vi "canDataSort.vi"() -> ()   [LabVIEW 2023] (continued)
 8        00\t00\tFF\tFF\tFF\tFF\tFF\tFF\r\n       712  1FFFFFFF   00000004    8        00\t20\tFF\tFF\tFF\tFF\tFF\tFF\r\n       703  0CF102A7   00000004    8        30\t75\tE0\t2E\t80\tFF\tFF\tFD\r\n       744  0CF103A7   00000004    8        17\t1F\t08\t60\tB1\t1F\t08\t3F\r\n       744  0CF102A7   00000004    8        30\t75\tE0\t2E\t80\tFF\tFF\tFD\r\n       743  0C3C4D4A   00000004    8        BE\tFF\tFF\t7F\t18\tFF\tFF\t3F\r\n       743  0CF101A7   00000004    8        68\t00\t97\tCC\t00\t15\t39\t3F\r\n       742  18F120F0   00000004    8        2B\t75\t60\tB1\tB0\t01\tFF\tFF\r\n       741  18F11FF0   00000004    8        FF\t3F\t90\t68\t88\t1B\t10\tFC\r\n       732  1FFFFFFF   00000004    8        00\t20\tFF\tFF\tFF\tFF\tFF\tFF\r\n       723  0CF102A7   00000004    8        30\t75\tE0\t2E\t80\tFF\tFF\tFD\r\n       723  0CF101A7   00000004    8        68\t00\t97\tCC\t00\t15\t39\t3E\r\n       722  1FFFFFFF   00000004    8        00\t00\tFF\tFF\tFF\tFF\tFF\tFF\r\n       712  1FFFFFFF   00000004    8        00\t20\tFF\tFF\tFF\tFF\tFF\tFF\r\n       745  0CF104A7   00000004    8        F0\t60\t22\tFC\tFF\tFF\tFF\t3F\r\n       744  0CF103A7   00000004    8        17\t1F\t08\t60\tB1\t1F\t08\t3F\r\n       744  0CF102A7   00000004    8        30\t75\tE0\t2E\t80\tFF\tFF\tFD\r\n       743  0C3C4D4A   00000004    8        BE\tFF\tFF\t7F\t18\tFF\tFF\t3F\r\n       743  0CF101A7   00000004    8        68\t00\t97\tCC\t00\t15\t39\t3F\r\n       742  18F120F0   00000004    8        2B\t75\t60\tB1\tB0\t01\tFF\tFF\r\n       741  18F11FF0   00000004    8        FF\t3F\t90\t68\t88\t1B\t10\tFC\r\n       732  1FFFFFFF   00000004    8        00\t20\tFF\tFF\tFF\tFF\tFF\tFF\r\n       723  0CF102A7   00000004    8        30\t75\tE0\t2E\t80\tFF\tFF\tFD\r\n       723  0CF101A7   00000004    8        68\t00\t97\tCC\t00\t15\t39\t3E\r\n       722  1FFFFFFF   00000004    8        00\t00\tFF\tFF\tFF\tFF\tFF\tFF\r\n       745  18F106A7   00000004    8        00\tF7\tFF\tFF\tFF\tFF\tFF\t7F\r\n       745  0CF104A7   00000004    8        F0\t60\t22\tFC\tFF\tFF\tFF\t3F\r\n       744  0CF103A7   00000004    8        17\t1F\t08\t60\tB1\t1F\t08\t3F\r\n       744  0CF102A7   00000004    8        30\t75\tE0\t2E\t80\tFF\tFF\tFD\r\n       743  0C3C4D4A   00000004    8        BE\tFF\tFF\t7F\t18\tFF\tFF\t3F\r\n       743  0CF101A7   00000004    8        68\t00\t97\tCC\t00\t15\t39\t3F\r\n       742  18F120F0   00000004    8        2B\t75\t60\tB1\tB0\t01\tFF\tFF\r\n       741  18F11FF0   00000004    8        FF\t3F\t90\t68\t88\t1B\t10\tFC\r\n       732  1FFFFFFF   00000004    8        00\t20\tFF\tFF\tFF\tFF\tFF\tFF\r\n       723  0CF102A7   00000004    8        30\t75\tE0\t2E\t80\tFF\tFF\tFD\r\n       723  0CF101A7   00000004    8        68\t00\t97\tCC\t00\t15\t39\t3E\r\n       746  18F121F0   00000004    8        09\t16\t00\t00\tFF\tFF\tB0\t01\r\n       745  18F106A7   00000004    8        00\tF7\tFF\tFF\tFF\tFF\tFF\t7F\r\n       745  0CF104A7   00000004    8        F0\t60\t22\tFC\tFF\tFF\tFF\t3F\r\n       744  0CF103A7   00000004    8        17\t1F\t08\t60\tB1\t1F\t08\t3F\r\n       744  0CF102A7   00000004    8        30\t75\tE0\t2E\t80\tFF\tFF\tFD\r\n       743  0C3C4D4A   00000004    8        BE\tFF\tFF\t7F\t18\tFF\tFF\t3F\r\n       743  0CF101A7   00000004    8        68\t00\t97\tCC\t00\t15\t39\t3F\r\n       742  18F120F0   00000004    8        2B\t75\t60\tB1\tB0\t01\tFF\tFF\r\n       741  18F11FF0   00000004    8        FF\t3F\t90\t68\t88\t1B\t10\tFC\r\n       732  1FFFFFFF   00000004    8        00\t20\tFF\tFF\tFF\tFF\tFF\tFF\r\n       723  0CF102A7   00000004    8        30\t75\tE0\t2E\t80\tFF\tFF\tFD\r\n       747  1FFFFFFF   00000004    8        00\t20\tFF\tFF\tFF\tFF\tFF\tFF\r\n       746  18F121F0   00000004    8        09\t16\t00\t00\tFF\tFF\tB0\t01\r\n       745  18F106A7   00000004    8        00\tF7\tFF\tFF\tFF\tFF\tFF\t7F\r\n       745  0CF104A7   00000004    8        F0\t60\t22\tFC\tFF\tFF\tFF\t3F\r\n       744  0CF103A7   00000004    8        17\t1F\t08\t60\tB1\t1F\t08\t3F\r\n       744  0CF102A7   00000004    8        30\t75\tE0\t2E\t80\tFF\tFF\tFD\r\n       743  0C3C4D4A   00000004    8        BE\tFF\tFF\t7F\t18\tFF\tFF\t3F\r\n       743  0CF101A7   00000004    8        68\t00\t97\tCC\t00\t15\t39\t3F\r\n       742  18F120F0   00000004    8        2B\t75\t60\tB1\tB0\t01\tFF\tFF\r\n       741  18F11FF0   00000004    8        FF\t3F\t90\t68\t88\t1B\t10\tFC\r\n       732  1FFFFFFF   00000004    8        00\t20\tFF\tFF\tFF\tFF\tFF\tFF\r\n       752  1FFFFFFF   00000004    8        00\t00\tFF\tFF\tFF\tFF\tFF\tFF\r\n       747  1FFFFFFF   00000004    8        00\t20\tFF\tFF\tFF\tFF\tFF\tFF\r\n       746  18F121F0   00000004    8        09\t16\t00\t00\tFF\tFF\tB0\t01\r\n       745  18F106A7   00000004    8        00\tF7\tFF\tFF\tFF\tFF\tFF\t7F\r\n       745  0CF104A7   00000004    8        F0\t60\t22\tFC\tFF\tFF\tFF\t3F\r\n       744  0CF103A7   00000004    8        17\t1F\t08\t60\tB1\t1F\t08\t3F\r\n       744  0CF102A7   00000004    8        30\t75\tE0\t2E\t80\tFF\tFF\tFD\r\n       743  0C3C4D4A   00000004    8        BE\tFF\tFF\t7F\t18\tFF\tFF\t3F\r\n       743  0CF101A7   00000004    8        68\t00\t97\tCC\t00\t15\t39\t3F\r\n       742  18F120F0   00000004    8        2B\t75\t60\tB1\tB0\t01\tFF\tFF\r\n       741  18F11FF0   00000004    8        FF\t3F\t90\t68\t88\t1B\t10\tFC\r\n       762  1FFFFFFF   00000004    8        00\t00\tFF\tFF\tFF\tFF\tFF\tFF\r\n       752  1FFFFFFF   00000004    8        00\t00\tFF\tFF\tFF\tFF\tFF\tFF\r\n       747  1FFFFFFF   00000004    8        00\t20\tFF\tFF\tFF\tFF\tFF\tFF\r\n       746  18F121F0   00000004    8        09\t16\t00\t00\tFF\tFF\tB0\t01\r\n       745  18F106A7   00000004    8        00\tF7\tFF\tFF\tFF\tFF\tFF\t7F\r\n       745  0CF104A7   00000004    8        F0\t60\t22\tFC\tFF\tFF\tFF\t3F\r\n       744  0CF103A7   00000004    8        17\t1F\t08\t60\tB1\t1F\t08\t3F\r\n       744  0CF102A7   00000004    8        30\t75\tE0\t2E\t80\tFF\tFF\tFD\r\n       743  0C3C4D4A   00000004    8        BE\tFF\tFF\t7F\t18\tFF\tFF\t3F\r\n       743  0CF101A7   00000004    8        68\t00\t97\tCC\t00\t15\t39\t3F\r\n       742  18F120F0   00000004    8        2B\t75\t60\tB1\tB0\t01\tFF\tFF\r\n       763  0CF101A7   00000004    8        68\t00\t97\tCC\t00\t15\t39\t40\r\n       762  1FFFFFFF   00000004    8        00\t00\tFF\tFF\tFF\tFF\tFF\tFF\r\n       752  1FFFFFFF   00000004    8        00\t00\tFF\tFF\tFF\tFF\tFF\tFF\r\n       747  1FFFFFFF   00000004    8        00\t20\tFF\tFF\tFF\tFF\tFF\tFF\r\n       746  18F121F0   00000004    8        09\t16\t00\t00\tFF\tFF\tB0\t01\r\n       745  18F106A7   00000004    8        00\tF7\tFF\tFF\tFF\tFF\tFF\t7F\r\n       745  0CF104A7   00000004    8        F0\t60\t22\tFC\tFF\tFF\tFF\t3F\r\n       744  0CF103A7   00000004    8        17\t1F\t08\t60\tB1\t1F\t08\t3F\r\n       744  0CF102A7   00000004    8        30\t75\tE0\t2E\t80\tFF\tFF\tFD\r\n       743  0C3C4D4A   00000004    8        BE\tFF\tFF\t7F\t18\tFF\tFF\t3F\r\n       743  0CF101A7   00000004    8        68\t00\t97\tCC\t00\t15\t39\t3F\r\n       763  0CF102A7   00000004    8        30\t75\tE0\t2E\t80\tFF\tFF\tFD\r\n       763  0CF101A7   00000004    8        68\t00\t97\tCC\t00\t15\t39\t40\r\n       762  1FFFFFFF   00000004    8        00\t00\tFF\tFF\tFF\tFF\tFF\tFF\r\n       752  1FFFFFFF   00000004    8        00\t00\tFF\tFF\tFF\tFF\tFF\tFF\r\n       747  1FFFFFFF   00000004    8        00\t20\tFF\tFF\tFF\tFF\tFF\tFF\r\n       746  18F121F0   00000004    8        09\t16\t00\t00\tFF\tFF\tB0\t01\r\n       745  18F106A7   00000004    8        00\tF7\tFF\tFF\tFF\tFF\tFF\t7F\r\n       745  0CF104A7   00000004    8        F0\t60\t22\tFC\tFF\tFF\tFF\t3F\r\n       744  0CF103A7   00000004    8        17\t1F\t08\t60\tB1\t1F\t08\t3F\r\n       744  0CF102A7   00000004    8        30\t75\tE0\t2E\t80\tFF\tFF\tFD\r\n       743  0C3C4D4A   00000004    8        BE\tFF\tFF\t7F\t18\tFF\tFF\t3F\r\n       772  1FFFFFFF   00000004    8        00\t00\tFF\tFF\tFF\tFF\tFF\tFF\r\n       763  0CF102A7   00000004    8        30\t75\tE0\t2E\t80\tFF\tFF\tFD\r\n       763  0CF101A7   00000004    8        68\t00\t97\tCC\t00\t15\t39\t40\r\n       762  1FFFFFFF   00000004    8        00\t00\tFF\tFF\tFF\tFF\tFF\tFF\r\n       752  1FFFFFFF   00000004    8        00\t00\tFF\tFF\tFF\tFF\tFF\tFF\r\n       747  1FFFFFFF   00000004    8        00\t20\tFF\tFF\tFF\tFF\tFF\tFF\r\n       746  18F121F0   00000004    8        09\t16\t00\t00\tFF\tFF\tB0\t01\r\n       745  18F106A7   00000004    8        00\tF7\tFF\tFF\tFF\tFF\tFF\t7F\r\n       745  0CF104A7   00000004    8        F0\t60\t22\tFC\tFF\tFF\tFF\t3F\r\n       744  0CF103A7   00000004    8        17\t1F\t08\t60\tB1\t1F\t08\t3F\r\n       744  0CF102A7   00000004    8        30\t75\tE0\t2E\t80\tFF\tFF\tFD\r\n       782  1FFFFFFF   00000004    8        00\t00\tFF\tFF\tFF\tFF\tFF\tFF\r\n       772  1FFFFFFF   00000004    8        00\t00\tFF\tFF\tFF\tFF\tFF\tFF\r\n       763  0CF102A7   00000004    8        30\t75\tE0\t2E\t80\tFF\tFF\tFD\r\n       763  0CF101A7   00000004    8        68\t00\t97\tCC\t00\t15\t39\t40\r\n       762  1FFFFFFF   00000004    8        00\t00\tFF\tFF\tFF\tFF\tFF\tFF\r\n       752  1FFFFFFF   00000004    8        00\t00\tFF\tFF\tFF\tFF\tFF\tFF\r\n       747  1FFFFFFF   00000004    8        00\t20\tFF\tFF\tFF\tFF\tFF\tFF\r\n       746  18F121F0   00000004    8        09\t16\t00\t00\tFF\tFF\tB0\t01\r\n       745  18F106A7   00000004    8        00\tF7\tFF\tFF\tFF\tFF\tFF\t7F\r\n       745  0CF104A7   00000004    8        F0\t60\t22\tFC\tFF\tFF\tFF\t3F\r\n       744  0CF103A7   00000004    8        17\t1F\t08\t60\tB1\t1F\t08\t3F\r\n       783  0CF101A7   00000004    8        68\t00\t97\tCC\t00\t15\t39\t41\r\n       782  1FFFFFFF   00000004    8        00\t00\tFF\tFF\tFF\tFF\tFF\tFF\r\n       772  1FFFFFFF   00000004    8        00\t00\tFF\tFF\tFF\tFF\tFF\tFF\r\n       763  0CF102A7   00000004    8        30\t75\tE0\t2E\t80\tFF\tFF\tFD\r\n       763  0CF101A7   00000004    8        68\t00\t97\tCC\t00\t15\t39\t40\r\n       762  1FFFFFFF   00000004    8        00\t00\tFF\tFF\tFF\tFF\tFF\tFF\r\n       752  1FFFFFFF   00000004    8        00\t00\tFF\tFF\tFF\tFF\tFF\tFF\r\n       747  1FFFFFFF   00000004    8        00\t20\tFF\tFF\tFF\tFF\tFF\tFF\r\n       746  18F121F0   00000004    8        09\t16\t00\t00\tFF\tFF\tB0\t01\r\n       745  18F106A7   00000004    8        00\tF7\tFF\tFF\tFF\tFF\tFF\t7F\r\n       745  0CF104A7   00000004    8        F0\t60\t22\tFC\tFF\tFF\tFF\t3F\r\n       783  0CF102A7   00000004    8        30\t75\tE0\t2E\t80\tFF\tFF\tFD\r\n       783  0CF101A7   00000004    8        68\t00\t97\tCC\t00\t15\t39\t41\r\n       782  1FFFFFFF   00000004    8        00\t00\tFF\tFF\tFF\tFF\tFF\tFF\r\n       772  1FFFFFFF   00000004    8        00\t00\tFF\tFF\tFF\tFF\tFF\tFF\r\n       763  0CF102A7   00000004    8        30\t75\tE0\t2E\t80\tFF\tFF\tFD\r\n       763  0CF101A7   00000004    8        68\t00\t97\tCC\t00\t15\t39\t40\r\n       762  1FFFFFFF   00000004    8        00\t00\tFF\tFF\tFF\tFF\tFF\tFF\r\n       752  1FFFFFFF   00000004    8        00\t00\tFF\tFF\tFF\tFF\tFF\tFF\r\n       747  1FFFFFFF   00000004    8        00\t20\tFF\tFF\tFF\tFF\tFF\tFF\r\n       746  18F121F0   00000004    8        09\t16\t00\t00\tFF\tFF\tB0\t01\r\n       745  18F106A7   00000004    8        00\tF7\tFF\tFF\tFF\tFF\tFF\t7F\r\n       792  1FFFFFFF   00000004    8        00\t20\tFF\tFF\tFF\tFF\tFF\tFF\r\n       783  0CF102A7   00000004    8        30\t75\tE0\t2E\t80\tFF\tFF\tFD\r\n       783  0CF101A7   00000004    8        68\t00\t97\tCC\t00\t15\t39\t41\r\n       782  1FFFFFFF   00000004    8        00\t00\tFF\tFF\tFF\tFF\tFF\tFF\r\n       772  1FFFFFFF   00000004    8        00\t00\tFF\tFF\tFF\tFF\tFF\tFF\r\n       763  0CF102A7   00000004    8        30\t75\tE0\t2E\t80\tFF\tFF\tFD\r\n       763  0CF101A7   00000004    8        68\t00\t97\tCC\t00\t15\t39\t40\r\n       762  1FFFFFFF   00000004    8        00\t00\tFF\tFF\tFF\tFF\tFF\tFF\r\n       752  1FFFFFFF   00000004    8        00\t00\tFF\tFF\tFF\tFF\tFF\tFF\r\n       747  1FFFFFFF   00000004    8        00\t20\tFF\tFF\tFF\tFF\tFF\tFF\r\n       746  18F121F0   00000004    8        09\t16\t00\t00\tFF\tFF\tB0\t01\r\n       793  18F106A7   00000004    8        00\tF7\tFF\tFF\tFF\tFF\tFF\t80\r\n       792  1FFFFFFF   00000004    8        00\t20\tFF\tFF\tFF\tFF\tFF\tFF\r\n       783  0CF102A7   00000004    8        30\t75\tE0\t2E\t80\tFF\tFF\tFD\r\n       783  0CF101A7   00000004    8        68\t00\t97\tCC\t00\t15\t39\t41\r\n       782  1FFFFFFF   00000004    8        00\t00\tFF\tFF\tFF\tFF\tFF\tFF\r\n       772  1FFFFFFF   00000004    8        00\t00\tFF\tFF\tFF\tFF\tFF\tFF\r\n       763  0CF102A7   00000004    8        30\t75\tE0\t2E\t80\tFF\tFF\tFD\r\n       763  0CF101A7   00000004    8        68\t00\t97\tCC\t00\t15\t39\t40\r\n       762  1FFFFFFF   00000004    8        00\t00\tFF\tFF\tFF\tFF\tFF\tFF\r\n       752  1FFFFFFF   00000004    8        00\t00\tFF\tFF\tFF\tFF\tFF\tFF\r\n       747  1FFFFFFF   00000004    8        00\t20\tFF\tFF\tFF\tFF\tFF\tFF\r\n       802  1FFFFFFF   00000004    8        00\t20\tFF\tFF\tFF\tFF\tFF\tFF\r\n       793  18F106A7   00000004    8        00\tF7\tFF\tFF\tFF\tFF\tFF\t80\r\n       792  1FFFFFFF   00000004    8        00\t20\tFF\tFF\tFF\tFF\tFF\tFF\r\n       783  0CF102A7   00000004    8        30\t75\tE0\t2E\t80\tFF\tFF\tFD\r\n       783  0CF101A7   00000004    8        68\t00\t97\tCC\t00\t15\t39\t41\r\n       782  1FFFFFFF   00000004    8        00\t00\tFF\tFF\tFF\tFF\tFF\tFF\r\n       772  1FFFFFFF   00000004    8        00\t00\tFF\tFF\tFF\tFF\tFF\tFF\r\n       763  0CF102A7   00000004    8        30\t75\tE0\t2E\t80\tFF\tFF\tFD\r\n       763  0CF101A7   00000004    8        68\t00\t97\tCC\t00\t15\t39\t40\r\n       762  1FFFFFFF   00000004    8        00\t00\tFF\tFF\tFF\tFF\tFF\tFF\r\n       752  1FFFFFFF   00000004    8        00\t00\tFF\tFF\tFF\tFF\tFF\tFF\r\n       803  0CF101A7   00000004    8        68\t00\t97\tCC\t00\t15\t39\t42\r\n       802  1FFFFFFF   00000004    8        00\t20\tFF\tFF\tFF\tFF\tFF\tFF\r\n       793  18F106A7   00000004    8        00\tF7\tFF\tFF\tFF\tFF\tFF\t80\r\n       792  1FFFFFFF   00000004    8        00\t20\tFF\tFF\tFF\tFF\tFF\tFF\r\n       783  0CF102A7   00000004    8        30\t75\tE0\t2E\t80\tFF\tFF\tFD\r\n       783  0CF101A7   00000004    8        68\t00\t97\tCC\t00\t15\t39\t41\r\n       782  1FFFFFFF   00000004    8        00\t00\tFF\tFF\tFF\tFF\tFF\tFF\r\n       772  1FFFFFFF   00000004    8        00\t00\tFF\tFF\tFF\tFF\tFF\tFF\r\n       763  0CF102A7   00000004    8        30\t75\tE0\t2E\t80\tFF\tFF\tFD\r\n       763  0CF101A7   00000004    8        68\t00\t97\tCC\t00\t15\t39\t40\r\n       762  1FFFFFFF   00000004    8        00\t00\tFF\tFF\tFF\tFF\tFF\tFF\r\n       803  0CF102A7   00000004    8        30\t75\tE0\t2E\t80\tFF\tFF\tFD\r\n       803  0CF101A7   00000004    8        68\t00\t97\tCC\t00\t15\t39\t42\r\n       802  1FFFFFFF   00000004    8        00\t20\tFF\tFF\tFF\tFF\tFF\tFF\r\n       793  18F106A7   00000004    8        00\tF7\tFF\tFF\tFF\tFF\tFF\t80\r\n       792  1FFFFFFF   00000004    8        00\t20\tFF\tFF\tFF\tFF\tFF\tFF\r\n       783  0CF102A7   00000004    8        30\t75\tE0\t2E\t80\tFF\tFF\tFD\r\n       783  0CF101A7   00000004    8        68\t00\t97\tCC\t00\t15\t39\t41\r\n       782  1FFFFFFF   00000004    8        00\t00\tFF\tFF\tFF\tFF\tFF\tFF\r\n       772  1FFFFFFF   00000004    8        00\t00\tFF\tFF\tFF\tFF\tFF\tFF\r\n       763  0CF102A7   00000004    8        30\t75\tE0\t2E\t80\tFF\tFF\tFD\r\n       763  0CF101A7   00000004    8        68\t00\t97\tCC\t00\t15\t39\t40\r\n       812  1FFFFFFF   00000004    8        00\t00\tFF\tFF\tFF\tFF\tFF\tFF\r\n       803  0CF102A7   00000004    8        30\t75\tE0\t2E\t80\tFF\tFF\tFD\r\n       803  0CF101A7   00000004    8        68\t00\t97\tCC\t00\t15\t39\t42\r\n       802  1FFFFFFF   00000004    8        00\t20\tFF\tFF\tFF\tFF\tFF\tFF\r\n       793  18F106A7   00000004    8        00\tF7\tFF\tFF\tFF\tFF\tFF\t80\r\n       792  1FFFFFFF   00000004    8        00\t20\tFF\tFF\tFF\tFF\tFF\tFF\r\n       783  0CF102A7   00000004    8        30\t75\tE0\t2E\t80\tFF\tFF\tFD\r\n       783  0CF101A7   00000004    8        68\t00\t97\tCC\t00\t15\t39\t41\r\n       782  1FFFFFFF   00000004    8        00\t00\tFF\tFF\tFF\tFF\tFF\tFF\r\n       772  1FFFFFFF   00000004    8        00\t00\tFF\tFF\tFF\tFF\tFF\tFF\r\n       763  0CF102A7   00000004    8        30\t75\tE0\t2E\t80\tFF\tFF\tFD\r\n       822  1FFFFFFF   00000004    8        00\t00\tFF\tFF\tFF\tFF\tFF\tFF\r\n       812  1FFFFFFF   00000004    8        00\t00\tFF\tFF\tFF\tFF\tFF\tFF\r\n       803  0CF102A7   00000004    8        30\t75\tE0\t2E\t80\tFF\tFF\tFD\r\n       803  0CF101A7   00000004    8        68\t00\t97\tCC\t00\t15\t39\t42\r\n       802  1FFFFFFF   00000004    8        00\t20\tFF\tFF\tFF\tFF\tFF\tFF\r\n       793  18F106A7   00000004    8        00\tF7\tFF\tFF\tFF\tFF\tFF\t80\r\n       792  1FFFFFFF   00000004    8        00\t20\tFF\tFF\tFF\tFF\tFF\tFF\r\n       783  0CF102A7   00000004    8        30\t75\tE0\t2E\t80\tFF\tFF\tFD\r\n       783  0CF101A7   00000004    8        68\t00\t97\tCC\t00\t15\t39\t41\r\n       782  1FFFFFFF   00000004    8        00\t00\tFF\tFF\tFF\tFF\tFF\tFF\r\n       772  1FFFFFFF   00000004    8        00\t00\tFF\tFF\tFF\tFF\tFF\tFF\r\n       823  0CF101A7   00000004    8        68\t00\t97\tCC\t00\t15\t39\t43\r\n       822  1FFFFFFF   00000004    8        00\t00\tFF\tFF\tFF\tFF\tFF\tFF\r\n       812  1FFFFFFF   00000004    8        00\t00\tFF\tFF\tFF\tFF\tFF\tFF\r\n       803  0CF102A7   00000004    8        30\t75\tE0\t2E\t80\tFF\tFF\tFD\r\n       803  0CF101A7   00000004    8        68\t00\t97\tCC\t00\t15\t39\t42\r\n       802  1FFFFFFF   00000004    8        00\t20\tFF\tFF\tFF\tFF\tFF\tFF\r\n       793  18F106A7   00000004    8        00\tF7\tFF\tFF\tFF\tFF\tFF\t80\r\n       792  1FFFFFFF   00000004    8        00\t20\tFF\tFF\tFF\tFF\tFF\tFF\r\n       783  0CF102A7   00000004    8        30\t75\tE0\t2E\t80\tFF\tFF\tFD\r\n       783  0CF101A7   00000004    8        68\t00\t97\tCC\t00\t15\t39\t41\r\n       782  1FFFFFFF   00000004    8        00\t00\tFF\tFF\tFF\tFF\tFF\tFF\r\n       823  0CF102A7   00000004    8        30\t75\tE0\t2E\t80\tFF\tFF\tFD\r\n       823  0CF101A7   00000004    8        68\t00\t97\tCC\t00\t15\t39\t43\r\n       822  1FFFFFFF   00000004    8        00\t00\tFF\tFF\tFF\tFF\tFF\tFF\r\n       812  1FFFFFFF   00000004    8        00\t00\tFF\tFF\tFF\tFF\tFF\tFF\r\n       803  0CF102A7   00000004    8        30\t75\tE0\t2E\t80\tFF\tFF\tFD\r\n       803  0CF101A7   00000004    8        68\t00\t97\tCC\t00\t15\t39\t42\r\n       802  1FFFFFFF   00000004    8        00\t20\tFF\tFF\tFF\tFF\tFF\tFF\r\n       793  18F106A7   00000004    8        00\tF7\tFF\tFF\tFF\tFF\tFF\t80\r\n       792  1FFFFFFF   00000004    8        00\t20\tFF\tFF\tFF\tFF\tFF\tFF\r\n       783  0CF102A7   00000004    8        30\t75\tE0\t2E\t80\tFF\tFF\tFD\r\n       783  0CF101A7   00000004    8        68\t00\t97\tCC\t00\t15\t39\t41\r\n       832  1FFFFFFF   00000004    8        00\t00\tFF\tFF\tFF\tFF\tFF\tFF\r\n       823  0CF102A7   00000004    8        30\t75\tE0\t2E\t80\tFF\tFF\tFD\r\n       823  0CF101A7   00000004    8        68\t00\t97\tCC\t00\t15\t39\t43\r\n       822  1FFFFFFF   00000004    8        00\t00\tFF\tFF\tFF\tFF\tFF\tFF\r\n       812  1FFFFFFF   00000004    8        00\t00\tFF\tFF\tFF\tFF\tFF\tFF\r\n       803  0CF102A7   00000004    8        30\t75\tE0\t2E\t80\tFF\tFF\tFD\r\n       803  0CF101A7   00000004    8        68\t00\t97\tCC\t00\t15\t39\t42\r\n       802  1FFFFFFF   00000004    8        00\t20\tFF\tFF\tFF\tFF\tFF\tFF\r\n       793  18F106A7   00000004    8        00\tF7\tFF\tFF\tFF\tFF\tFF\t80\r\n       792  1FFFFFFF   00000004    8        00\t20\tFF\tFF\tFF\tFF\tFF\tFF\r\n       783  0CF102A7   00000004    8        30\t75\tE0\t2E\t80\tFF\tFF\tFD\r\n       841  18F11FF0   00000004    8        FF\t3F\t90\t68\t88\t1B\t10\t0C\r\n       832  1FFFFFFF   00000004    8        00\t00\tFF\tFF\tFF\tFF\tFF\tFF\r\n       823  0CF102A7   00000004    8        30\t75\tE0\t2E\t80\tFF\tFF\tFD\r\n       823  0CF101A7   00000004    8        68\t00\t97\tCC\t00\t15\t39\t43\r\n       822  1FFFFFFF   00000004    8        00\t00\tFF\tFF\tFF\tFF\tFF\tFF\r\n       812  1FFFFFFF   00000004    8        00\t00\tFF\tFF\tFF\tFF\tFF\tFF\r\n       803  0CF102A7   00000004    8        30\t75\tE0\t2E\t80\tFF\tFF\tFD\r\n       803  0CF101A7   00000004    8        68\t00\t97\tCC\t00\t15\t39\t42\r\n       802  1FFFFFFF   00000004    8        00\t20\tFF\tFF\tFF\tFF\tFF\tFF\r\n       793  18F106A7   00000004    8        00\tF7\tFF\tFF\tFF\tFF\tFF\t80\r\n       792  1FFFFFFF   00000004    8        00\t20\tFF\tFF\tFF\tFF\tFF\tFF\r\n       842  18F120F0   00000004    8        2B\t75\t60\tB1\tB0\t01\tFF\tFF\r\n       841  18F11FF0   00000004    8        FF\t3F\t90\t68\t88\t1B\t10\t0C\r\n       832  1FFFFFFF   00000004    8        00\t00\tFF\tFF\tFF\tFF\tFF\tFF\r\n       823  0CF102A7   00000004    8        30\t75\tE0\t2E\t80\tFF\tFF\tFD\r\n       823  0CF101A7   00000004    8        68\t00\t97\tCC\t00\t15\t39\t43\r\n       822  1FFFFFFF   00000004    8        00\t00\tFF\tFF\tFF\tFF\tFF\tFF\r\n       812  1FFFFFFF   00000004    8        00\t00\tFF\tFF\tFF\tFF\tFF\tFF\r\n       803  0CF102A7   00000004    8        30\t75\tE0\t2E\t80\tFF\tFF\tFD\r\n       803  0CF101A7   00000004    8        68\t00\t97\tCC\t00\t15\t39\t42\r\n       802  1FFFFFFF   00000004    8        00\t20\tFF\tFF\tFF\tFF\tFF\tFF\r\n       793  18F106A7   00000004    8        00\tF7\tFF\tFF\tFF\tFF\tFF\t80\r\n       843  0CF101A7   00000004    8        68\t00\t97\tCC\t00\t15\t39\t44\r\n       842  18F120F0   00000004    8        2B\t75\t60\tB1\tB0\t01\tFF\tFF\r\n       841  18F11FF0   00000004    8        FF\t3F\t90\t68\t88\t1B\t10\t0C\r\n       832  1FFFFFFF   00000004    8        00\t00\tFF\tFF\tFF\tFF\tFF\tFF\r\n       823  0CF102A7   00000004    8        30\t75\tE0\t2E\t80\tFF\tFF\tFD\r\n       823  0CF101A7   00000004    8        68\t00\t97\tCC\t00\t15\t39\t43\r\n       822  1FFFFFFF   00000004    8        00\t00\tFF\tFF\tFF\tFF\tFF\tFF\r\n       812  1FFFFFFF   00000004    8        00\t00\tFF\tFF\tFF\tFF\tFF\tFF\r\n       803  0CF102A7   00000004    8        30\t75\tE0\t2E\t80\tFF\tFF\tFD\r\n       803  0CF101A7   00000004    8        68\t00\t97\tCC\t00\t15\t39\t42\r\n       802  1FFFFFFF   00000004    8        00\t20\tFF\tFF\tFF\tFF\tFF\tFF\r\n       843  0C3C4D4A   00000004    8        BE\tFF\tFF\t7F\t18\tFF\tFF\t40\r\n       843  0CF101A7   00000004    8        68\t00\t97\tCC\t00\t15\t39\t44\r\n       842  18F120F0   00000004    8        2B\t75\t60\tB1\tB0\t01\tFF\tFF\r\n       841  18F11FF0   00000004    8        FF\t3F\t90\t68\t88\t1B\t10\t0C\r\n       832  1FFFFFFF   00000004    8        00\t00\tFF\tFF\tFF\tFF\tFF\tFF\r\n       823  0CF102A7   00000004    8        30\t75\tE0\t2E\t80\tFF\tFF\tFD\r\n       823  0CF101A7   00000004    8        68\t00\t97\tCC\t00\t15\t39\t43\r\n       822  1FFFFFFF   00000004    8        00\t00\tFF\tFF\tFF\tFF\tFF\tFF\r\n       812  1FFFFFFF   00000004    8        00\t00\tFF\tFF\tFF\tFF\tFF\tFF\r\n       803  0CF102A7   00000004    8        30\t75\tE0\t2E\t80\tFF\tFF\tFD\r\n       803  0CF101A7   00000004    8        68\t00\t97\tCC\t00\t15\t39\t42\r\n       844  0CF102A7   00000004    8        30\t75\tE0\t2E\t80\tFF\tFF\tFD\r\n       843  0C3C4D4A   00000004    8        BE\tFF\tFF\t7F\t18\tFF\tFF\t40\r\n       843  0CF101A7   00000004    8        68\t00\t97\tCC\t00\t15\t39\t44\r\n       842  18F120F0   00000004    8        2B\t75\t60\tB1\tB0\t01\tFF\tFF\r\n       841  18F11FF0   00000004    8        FF\t3F\t90\t68\t88\t1B\t10\t0C\r\n       832  1FFFFFFF   00000004    8        00\t00\tFF\tFF\tFF\tFF\tFF\tFF\r\n       823  0CF102A7   00000004    8        30\t75\tE0\t2E\t80\tFF\tFF\tFD\r\n       823  0CF101A7   00000004    8        68\t00\t97\tCC\t00\t15\t39\t43\r\n       822  1FFFFFFF   00000004    8        00\t00\tFF\tFF\tFF\tFF\tFF\tFF\r\n       812  1FFFFFFF   00000004    8        00\t00\tFF\tFF\tFF\tFF\tFF\tFF\r\n       803  0CF102A7   00000004    8        30\t75\tE0\t2E\t80\tFF\tFF\tFD\r\n       844  0CF103A7   00000004    8        17\t1F\t08\t60\tB1\t1F\t08\t40\r\n       844  0CF102A7   00000004    8        30\t75\tE0\t2E\t80\tFF\tFF\tFD\r\n       843  0C3C4D4A   00000004    8        BE\tFF\tFF\t7F\t18\tFF\tFF\t40\r\n       843  0CF101A7   00000004    8        68\t00\t97\tCC\t00\t15\t39\t44\r\n       842  18F120F0   00000004    8        2B\t75\t60\tB1\tB0\t01\tFF\tFF\r\n       841  18F11FF0   00000004    8        FF\t3F\t90\t68\t88\t1B\t10\t0C\r\n       832  1FFFFFFF   00000004    8        00\t00\tFF\tFF\tFF\tFF\tFF\tFF\r\n       823  0CF102A7   00000004    8        30\t75\tE0\t2E\t80\tFF\tFF\tFD\r\n       823  0CF101A7   00000004    8        68\t00\t97\tCC\t00\t15\t39\t43\r\n       822  1FFFFFFF   00000004    8        00\t00\tFF\tFF\tFF\tFF\tFF\tFF\r\n       812  1FFFFFFF   00000004    8        00\t00\tFF\tFF\tFF\tFF\tFF\tFF\r\n       845  0CF104A7   00000004    8        F0\t60\t22\tFC\tFF\tFF\tFF\t40\r\n       844  0CF103A7   00000004    8        17\t1F\t08\t60\tB1\t1F\t08\t40\r\n       844  0CF102A7   00000004    8        30\t75\tE0\t2E\t80\tFF\tFF\tFD\r\n       843  0C3C4D4A   00000004    8        BE\tFF\tFF\t7F\t18\tFF\tFF\t40\r\n       843  0CF101A7   00000004    8        68\t00\t97\tCC\t00\t15\t39\t44\r\n       842  18F120F0   00000004    8        2B\t75\t60\tB1\tB0\t01\tFF\tFF\r\n       841  18F11FF0   00000004    8        FF\t3F\t90\t68\t88\t1B\t10\t0C\r\n       832  1FFFFFFF   00000004    8        00\t00\tFF\tFF\tFF\tFF\tFF\tFF\r\n       823  0CF102A7   00000004    8        30\t75\tE0\t2E\t80\tFF\tFF\tFD\r\n       823  0CF101A7   00000004    8        68\t00\t97\tCC\t00\t15\t39\t43\r\n       822  1FFFFFFF   00000004    8        00\t00\tFF\tFF\tFF\tFF\tFF\tFF\r\n       846  18F106A7   00000004    8        00\tF7\tFF\tFF\tFF\tFF\tFF\t81\r\n       845  0CF104A7   00000004    8        F0\t60\t22\tFC\tFF\tFF\tFF\t40\r\n       844  0CF103A7   00000004    8        17\t1F\t08\t60\tB1\t1F\t08\t40\r\n       844  0CF102A7   00000004    8        30\t75\tE0\t2E\t80\tFF\tFF\tFD\r\n       843  0C3C4D4A   00000004    8        BE\tFF\tFF\t7F\t18\tFF\tFF\t40\r\n       843  0CF101A7   00000004    8        68\t00\t97\tCC\t00\t15\t39\t44\r\n       842  18F120F0   00000004    8        2B\t75\t60\tB1\tB0\t01\tFF\tFF\r\n       841  18F11FF0   00000004    8        FF\t3F\t90\t68\t88\t1B\t10\t0C\r\n       832  1FFFFFFF   00000004    8        00\t00\tFF\tFF\tFF\tFF\tFF\tFF\r\n       823  0CF102A7   00000004    8        30\t75\tE0\t2E\t80\tFF\tFF\tFD\r\n       823  0CF101A7   00000004    8        68\t00\t97\tCC\t00\t15\t39\t43\r\n       846  18F121F0   00000004    8        09\t16\t00\t00\tFF\tFF\tB0\t01\r\n       846  18F106A7   00000004    8        00\tF7\tFF\tFF\tFF\tFF\tFF\t81\r\n       845  0CF104A7   00000004    8        F0\t60\t22\tFC\tFF\tFF\tFF\t40\r\n       844  0CF103A7   00000004    8        17\t1F\t08\t60\tB1\t1F\t08\t40\r\n       844  0CF102A7   00000004    8        30\t75\tE0\t2E\t80\tFF\tFF\tFD\r\n       843  0C3C4D4A   00000004    8        BE\tFF\tFF\t7F\t18\tFF\tFF\t40\r\n       843  0CF101A7   00000004    8        68\t00\t97\tCC\t00\t15\t39\t44\r\n       842  18F120F0   00000004    8        2B\t75\t60\tB1\tB0\t01\tFF\tFF\r\n       841  18F11FF0   00000004    8        FF\t3F\t90\t68\t88\t1B\t10\t0C\r\n       832  1FFFFFFF   00000004    8        00\t00\tFF\tFF\tFF\tFF\tFF\tFF\r\n       823  0CF102A7   00000004    8        30\t75\tE0\t2E\t80\tFF\tFF\tFD\r\n       847  1FFFFFFF   00000004    8        00\t00\tFF\tFF\tFF\tFF\tFF\tFF\r\n       846  18F121F0   00000004    8        09\t16\t00\t00\tFF\tFF\tB0\t01\r\n       846  18F106A7   00000004    8        00\tF7\tFF\tFF\tFF\tFF\tFF\t81\r\n       845  0CF104A7   00000004    8        F0\t60\t22\tFC\tFF\tFF\tFF\t40\r\n       844  0CF103A7   00000004    8        17\t1F\t08\t60\tB1\t1F\t08\t40\r\n       844  0CF102A7   00000004    8        30\t75\tE0\t2E\t80\tFF\tFF\tFD\r\n       843  0C3C4D4A   00000004    8        BE\tFF\tFF\t7F\t18\tFF\tFF\t40\r\n       843  0CF101A7   00000004    8        68\t00\t97\tCC\t00\t15\t39\t44\r\n       842  18F120F0   00000004    8        2B\t75\t60\tB1\tB0\t01\tFF\tFF\r\n       841  18F11FF0   00000004    8        FF\t3F\t90\t68\t88\t1B\t10\t0C\r\n       832  1FFFFFFF   00000004    8        00\t00\tFF\tFF\tFF\tFF\tFF\tFF\r\n       852  1FFFFFFF   00000004    8        00\t00\tFF\tFF\tFF\tFF\tFF\tFF\r\n       847  1FFFFFFF   00000004    8        00\t00\tFF\tFF\tFF\tFF\tFF\tFF\r\n       846  18F121F0   00000004    8        09\t16\t00\t00\tFF\tFF\tB0\t01\r\n       846  18F106A7   00000004    8        00\tF7\tFF\tFF\tFF\tFF\tFF\t81\r\n       845  0CF104A7   00000004    8        F0\t60\t22\tFC\tFF\tFF\tFF\t40\r\n       844  0CF103A7   00000004    8        17\t1F\t08\t60\tB1\t1F\t08\t40\r\n       844  0CF102A7   00000004    8        30\t75\tE0\t2E\t80\tFF\tFF\tFD\r\n       843  0C3C4D4A   00000004    8        BE\tFF\tFF\t7F\t18\tFF\tFF\t40\r\n       843  0CF101A7   00000004    8        68\t00\t97\tCC\t00\t15\t39\t44\r\n       842  18F120F0   00000004    8        2B\t75\t60\tB1\tB0\t01\tFF\tFF\r\n       841  18F11FF0   00000004    8        FF\t3F\t90\t68\t88\t1B\t10\t0C\r\n       862  1FFFFFFF   00000004    8        00\t00\tFF\tFF\tFF\tFF\tFF\tFF\r\n       852  1FFFFFFF   00000004    8        00\t00\tFF\tFF\tFF\tFF\tFF\tFF\r\n       847  1FFFFFFF   00000004    8        00\t00\tFF\tFF\tFF\tFF\tFF\tFF\r\n       846  18F121F0   00000004    8        09\t16\t00\t00\tFF\tFF\tB0\t01\r\n       846  18F106A7   00000004    8        00\tF7\tFF\tFF\tFF\tFF\tFF\t81\r\n       845  0CF104A7   00000004    8        F0\t60\t22\tFC\tFF\tFF\tFF\t40\r\n       844  0CF103A7   00000004    8        17\t1F\t08\t60\tB1\t1F\t08\t40\r\n       844  0CF102A7   00000004    8        30\t75\tE0\t2E\t80\tFF\tFF\tFD\r\n       843  0C3C4D4A   00000004    8        BE\tFF\tFF\t7F\t18\tFF\tFF\t40\r\n       843  0CF101A7   00000004    8        68\t00\t97\tCC\t00\t15\t39\t44\r\n       842  18F120F0   00000004    8        2B\t75\t60\tB1\tB0\t01\tFF\tFF\r\n       863  0CF101A7   00000004    8        68\t00\t97\tCC\t00\t15\t39\t45\r\n       862  1FFFFFFF   00000004    8        00\t00\tFF\tFF\tFF\tFF\tFF\tFF\r\n       852  1FFFFFFF   00000004    8        00\t00\tFF\tFF\tFF\tFF\tFF\tFF\r\n       847  1FFFFFFF   00000004    8        00\t00\tFF\tFF\tFF\tFF\tFF\tFF\r\n       846  18F121F0   00000004    8        09\t16\t00\t00\tFF\tFF\tB0\t01\r\n       846  18F106A7   00000004    8        00\tF7\tFF\tFF\tFF\tFF\tFF\t81\r\n       845  0CF104A7   00000004    8        F0\t60\t22\tFC\tFF\tFF\tFF\t40\r\n       844  0CF103A7   00000004    8        17\t1F\t08\t60\tB1\t1F\t08\t40\r\n       844  0CF102A7   00000004    8        30\t75\tE0\t2E\t80\tFF\tFF\tFD\r\n       843  0C3C4D4A   00000004    8        BE\tFF\tFF\t7F\t18\tFF\tFF\t40\r\n       843  0CF101A7   00000004    8        68\t00\t97\tCC\t00\t15\t39\t44\r\n       863  0CF102A7   00000004    8        30\t75\tE0\t2E\t80\tFF\tFF\tFD\r\n       863  0CF101A7   00000004    8        68\t00\t97\tCC\t00\t15\t39\t45\r\n       862  1FFFFFFF   00000004    8        00\t00\tFF\tFF\tFF\tFF\tFF\tFF\r\n       852  1FFFFFFF   00000004    8        00\t00\tFF\tFF\tFF\tFF\tFF\tFF\r\n       847  1FFFFFFF   00000004    8        00\t00\tFF\tFF\tFF\tFF\tFF\tFF\r\n       846  18F121F0   00000004    8        09\t16\t00\t00\tFF\tFF\tB0\t01\r\n       846  18F106A7   00000004    8        00\tF7\tFF\tFF\tFF\tFF\tFF\t81\r\n       845  0CF104A7   00000004    8        F0\t60\t22\tFC\tFF\tFF\tFF\t40\r\n       844  0CF103A7   00000004    8        17\t1F\t08\t60\tB1\t1F\t08\t40\r\n       844  0CF102A7   00000004    8        30\t75\tE0\t2E\t80\tFF\tFF\tFD\r\n       843  0C3C4D4A   00000004    8        BE\tFF\tFF\t7F\t18\tFF\tFF\t40\r\n       872  1FFFFFFF   00000004    8        00\t00\tFF\tFF\tFF\tFF\tFF\tFF\r\n       863  0CF102A7   00000004    8        30\t75\tE0\t2E\t80\tFF\tFF\tFD\r\n       863  0CF101A7   00000004    8        68\t00\t97\tCC\t00\t15\t39\t45\r\n       862  1FFFFFFF   00000004    8        00\t00\tFF\tFF\tFF\tFF\tFF\tFF\r\n       852  1FFFFFFF   00000004    8        00\t00\tFF\tFF\tFF\tFF\tFF\tFF\r\n       847  1FFFFFFF   00000004    8        00\t00\tFF\tFF\tFF\tFF\tFF\tFF\r\n       846  18F121F0   00000004    8        09\t16\t00\t00\tFF\tFF\tB0\t01\r\n       846  18F106A7   00000004    8        00\tF7\tFF\tFF\tFF\tFF\tFF\t81\r\n       845  0CF104A7   00000004    8        F0\t60\t22\tFC\tFF\tFF\tFF\t40\r\n       844  0CF103A7   00000004    8        17\t1F\t08\t60\tB1\t1F\t08\t40\r\n       844  0CF102A7   00000004    8        30\t75\tE0\t2E\t80\tFF\tFF\tFD\r\n       882  1FFFFFFF   00000004    8        00\t00\tFF\tFF\tFF\tFF\tFF\tFF\r\n       872  1FFFFFFF   00000004    8        00\t00\tFF\tFF\tFF\tFF\tFF\tFF\r\n       863  0CF102A7   00000004    8        30\t75\tE0\t2E\t80\tFF\tFF\tFD\r\n       863  0CF101A7   00000004    8        68\t00\t97\tCC\t00\t15\t39\t45\r\n       862  1FFFFFFF   00000004    8        00\t00\tFF\tFF\tFF\tFF\tFF\tFF\r\n       852  1FFFFFFF   00000004    8        00\t00\tFF\tFF\tFF\tFF\tFF\tFF\r\n       847  1FFFFFFF   00000004    8        00\t00\tFF\tFF\tFF\tFF\tFF\tFF\r\n       846  18F121F0   00000004    8        09\t16\t00\t00\tFF\tFF\tB0\t01\r\n       846  18F106A7   00000004    8        00\tF7\tFF\tFF\tFF\tFF\tFF\t81\r\n       845  0CF104A7   00000004    8        F0\t60\t22\tFC\tFF\tFF\tFF\t40\r\n       844  0CF103A7   00000004    8        17\t1F\t08\t60\tB1\t1F\t08\t40\r\n       883  0CF101A7   00000004    8        68\t00\t97\tCC\t00\t15\t39\t46\r\n       882  1FFFFFFF   00000004    8        00\t00\tFF\tFF\tFF\tFF\tFF\tFF\r\n       872  1FFFFFFF   00000004    8        00\t00\tFF\tFF\tFF\tFF\tFF\tFF\r\n       863  0CF102A7   00000004    8        30\t75\tE0\t2E\t80\tFF\tFF\tFD\r\n       863  0CF101A7   00000004    8        68\t00\t97\tCC\t00\t15\t39\t45\r\n       862  1FFFFFFF   00000004    8        00\t00\tFF\tFF\tFF\tFF\tFF\tFF\r\n       852  1FFFFFFF   00000004    8        00\t00\tFF\tFF\tFF\tFF\tFF\tFF\r\n       847  1FFFFFFF   00000004    8        00\t00\tFF\tFF\tFF\tFF\tFF\tFF\r\n       846  18F121F0   00000004    8        09\t16\t00\t00\tFF\tFF\tB0\t01\r\n       846  18F106A7   00000004    8        00\tF7\tFF\tFF\tFF\tFF\tFF\t81\r\n       845  0CF104A7   00000004    8        F0\t60\t22\tFC\tFF\tFF\tFF\t40\r\n       883  0CF102A7   00000004    8        30\t75\tE0\t2E\t80\tFF\tFF\tFD\r\n       883  0CF101A7   00000004    8        68\t00\t97\tCC\t00\t15\t39\t46\r\n       882  1FFFFFFF   00000004    8        00\t00\tFF\tFF\tFF\tFF\tFF\tFF\r\n       872  1FFFFFFF   00000004    8        00\t00\tFF\tFF\tFF\tFF\tFF\tFF\r\n       863  0CF102A7   00000004    8        30\t75\tE0\t2E\t80\tFF\tFF\tFD\r\n       863  0CF101A7   00000004    8        68\t00\t97\tCC\t00\t15\t39\t45\r\n       862  1FFFFFFF   00000004    8        00\t00\tFF\tFF\tFF\tFF\tFF\tFF\r\n       852  1FFFFFFF   00000004    8        00\t00\tFF\tFF\tFF\tFF\tFF\tFF\r\n       847  1FFFFFFF   00000004    8        00\t00\tFF\tFF\tFF\tFF\tFF\tFF\r\n       846  18F121F0   00000004    8        09\t16\t00\t00\tFF\tFF\tB0\t01\r\n       846  18F106A7   00000004    8        00\tF7\tFF\tFF\tFF\tFF\tFF\t81\r\n       892  1FFFFFFF   00000004    8        00\t00\tFF\tFF\tFF\tFF\tFF\tFF\r\n       883  0CF102A7   00000004    8        30\t75\tE0\t2E\t80\tFF\tFF\tFD\r\n       883  0CF101A7   00000004    8        68\t00\t97\tCC\t00\t15\t39\t46\r\n       882  1FFFFFFF   00000004    8        00\t00\tFF\tFF\tFF\tFF\tFF\tFF\r\n       872  1FFFFFFF   00000004    8        00\t00\tFF\tFF\tFF\tFF\tFF\tFF\r\n       863  0CF102A7   00000004    8        30\t75\tE0\t2E\t80\tFF\tFF\tFD\r\n       863  0CF101A7   00000004    8        68\t00\t97\tCC\t00\t15\t39\t45\r\n       862  1FFFFFFF   00000004    8        00\t00\tFF\tFF\tFF\tFF\tFF\tFF\r\n       852  1FFFFFFF   00000004    8        00\t00\tFF\tFF\tFF\tFF\tFF\tFF\r\n       847  1FFFFFFF   00000004    8        00\t00\tFF\tFF\tFF\tFF\tFF\tFF\r\n       846  18F121F0   00000004    8        09\t16\t00\t00\tFF\tFF\tB0\t01\r\n       893  18F106A7   00000004    8        00\tF7\tFF\tFF\tFF\tFF\tFF\t82\r\n       892  1FFFFFFF   00000004    8        00\t00\tFF\tFF\tFF\tFF\tFF\tFF\r\n       883  0CF102A7   00000004    8        30\t75\tE0\t2E\t80\tFF\tFF\tFD\r\n       883  0CF101A7   00000004    8        68\t00\t97\tCC\t00\t15\t39\t46\r\n       882  1FFFFFFF   00000004    8        00\t00\tFF\tFF\tFF\tFF\tFF\tFF\r\n       872  1FFFFFFF   00000004    8        00\t00\tFF\tFF\tFF\tFF\tFF\tFF\r\n       863  0CF102A7   00000004    8        30\t75\tE0\t2E\t80\tFF\tFF\tFD\r\n       863  0CF101A7   00000004    8        68\t00\t97\tCC\t00\t15\t39\t45\r\n       862  1FFFFFFF   00000004    8        00\t00\tFF\tFF\tFF\tFF\tFF\tFF\r\n       852  1FFFFFFF   00000004    8        00\t00\tFF\tFF\tFF\tFF\tFF\tFF\r\n       847  1FFFFFFF   00000004    8        00\t00\tFF\tFF\tFF\tFF\tFF\tFF\r\n       902  1FFFFFFF   00000004    8        00\t00\tFF\tFF\tFF\tFF\tFF\tFF\r\n       893  18F106A7   00000004    8        00\tF7\tFF\tFF\tFF\tFF\tFF\t82\r\n       892  1FFFFFFF   00000004    8        00\t00\tFF\tFF\tFF\tFF\tFF\tFF\r\n       883  0CF102A7   00000004    8        30\t75\tE0\t2E\t80\tFF\tFF\tFD\r\n       883  0CF101A7   00000004    8        68\t00\t97\tCC\t00\t15\t39\t46\r\n       882  1FFFFFFF   00000004    8        00\t00\tFF\tFF\tFF\tFF\tFF\tFF\r\n       872  1FFFFFFF   00000004    8        00\t00\tFF\tFF\tFF\tFF\tFF\tFF\r\n       863  0CF102A7   00000004    8        30\t75\tE0\t2E\t80\tFF\tFF\tFD\r\n       863  0CF101A7   00000004    8        68\t00\t97\tCC\t00\t15\t39\t45\r\n       862  1FFFFFFF   00000004    8        00\t00\tFF\tFF\tFF\tFF\tFF\tFF\r\n       852  1FFFFFFF   00000004    8        00\t00\tFF\tFF\tFF\tFF\tFF\tFF\r\n       903  0CF101A7   00000004    8        68\t00\t97\tCC\t00\t15\t39\t47\r\n       902  1FFFFFFF   00000004    8        00\t00\tFF\tFF\tFF\tFF\tFF\tFF\r\n       893  18F106A7   00000004    8        00\tF7\tFF\tFF\tFF\tFF\tFF\t82\r\n       892  1FFFFFFF   00000004    8        00\t00\tFF\tFF\tFF\tFF\tFF\tFF\r\n       883  0CF102A7   00000004    8        30\t75\tE0\t2E\t80\tFF\tFF\tFD\r\n       883  0CF101A7   00000004    8        68\t00\t97\tCC\t00\t15\t39\t46\r\n       882  1FFFFFFF   00000004    8        00\t00\tFF\tFF\tFF\tFF\tFF\tFF\r\n       872  1FFFFFFF   00000004    8        00\t00\tFF\tFF\tFF\tFF\tFF\tFF\r\n       863  0CF102A7   00000004    8        30\t75\tE0\t2E\t80\tFF\tFF\tFD\r\n       863  0CF101A7   00000004    8        68\t00\t97\tCC\t00\t15\t39\t45\r\n       862  1FFFFFFF   00000004    8        00\t00\tFF\tFF\tFF\tFF\tFF\tFF\r\n       903  0CF102A7   00000004    8        30\t75\tE0\t2E\t80\tFF\tFF\tFD\r\n       903  0CF101A7   00000004    8        68\t00\t97\tCC\t00\t15\t39\t47\r\n       902  1FFFFFFF   00000004    8        00\t00\tFF\tFF\tFF\tFF\tFF\tFF\r\n       893  18F106A7   00000004    8        00\tF7\tFF\tFF\tFF\tFF\tFF\t82\r\n       892  1FFFFFFF   00000004    8        00\t00\tFF\tFF\tFF\tFF\tFF\tFF\r\n       883  0CF102A7   00000004    8        30\t75\tE0\t2E\t80\tFF\tFF\tFD\r\n       883  0CF101A7   00000004    8        68\t00\t97\tCC\t00\t15\t39\t46\r\n       882  1FFFFFFF   00000004    8        00\t00\tFF\tFF\tFF\tFF\tFF\tFF\r\n       872  1FFFFFFF   00000004    8        00\t00\tFF\tFF\tFF\tFF\tFF\tFF\r\n       863  0CF102A7   00000004    8        30\t75\tE0\t2E\t80\tFF\tFF\tFD\r\n       863  0CF101A7   00000004    8        68\t00\t97\tCC\t00\t15\t39\t45\r\n       912  1FFFFFFF   00000004    8        00\t00\tFF\tFF\tFF\tFF\tFF\tFF\r\n       903  0CF102A7   00000004    8        30\t75\tE0\t2E\t80\tFF\tFF\tFD\r\n       903  0CF101A7   00000004    8        68\t00\t97\tCC\t00\t15\t39\t47\r\n       902  1FFFFFFF   00000004    8        00\t00\tFF\tFF\tFF\tFF\tFF\tFF\r\n       893  18F106A7
